vi "Cost.vi"(8 "error in (no error)":errorcluster, 11 "Whip in":refnum<class "Whip.lvclass">) -> (0 "error out":errorcluster, 2 "Cost":dbl, 3 "Whip out":refnum<class "Whip.lvclass">)   [LabVIEW 2011, in "Whip.lvclass"]
uses:
  Whip.lvclass
  Whip.lvclass/Whip.ctl
  Beverage/Beverage.lvclass
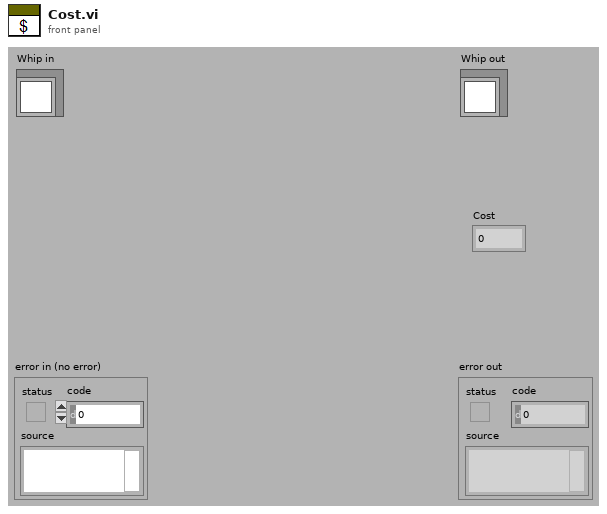
[diagram p1: front panel]
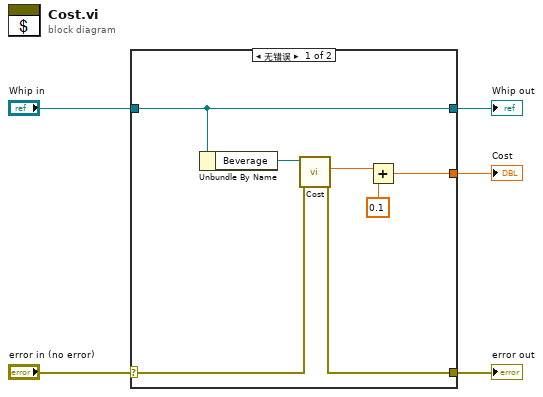
[diagram p0: block diagram]
diagram:
  n1 = case shown="无错误" "error in (no error)" {
    selector: "error in (no error)" -> [w10 w14]
    tunnel: [w9 w14] -> w4
    tunnel: [w12 w13] -> w2
    tunnel: "Whip in" -> [w12 w13]
    tunnel: [w6 _] -> w1
    frame No Error {
      n2 = Unbundle By Name(w12) -> ("Beverage"=w11:refnum<class "Beverage.lvclass">)
      n3 = call-dynamic "Cost.vi"("error in (no error)"=w10, "Beverage in"=w11) -> ("error out"=w9:errorcluster, "Cost"=w8:dbl)  [unwired: 7 in, 1 out]
      n4 = Add(x=w8, y=0.1) -> (x+y=w6:dbl)
    }
    frame Error {
    }
  }
  "error out" <- w4
  "Whip out" <- w2
  "Cost" <- w1
